vi "Auto 9.vi"(8 "Error In":errorcluster) -> (0 "Error Out":errorcluster)   [LabVIEW 2014]
uses:
  <vilib>/Rock Robotics/Network Tables/SD Read Boolean.vi
  Global Variables/Refnum Names.vi
  <vilib>/Rock Robotics/Network Tables/SD Read Number.vi
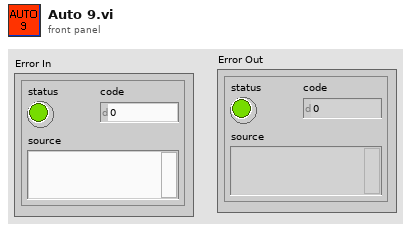
[diagram p1: front panel]
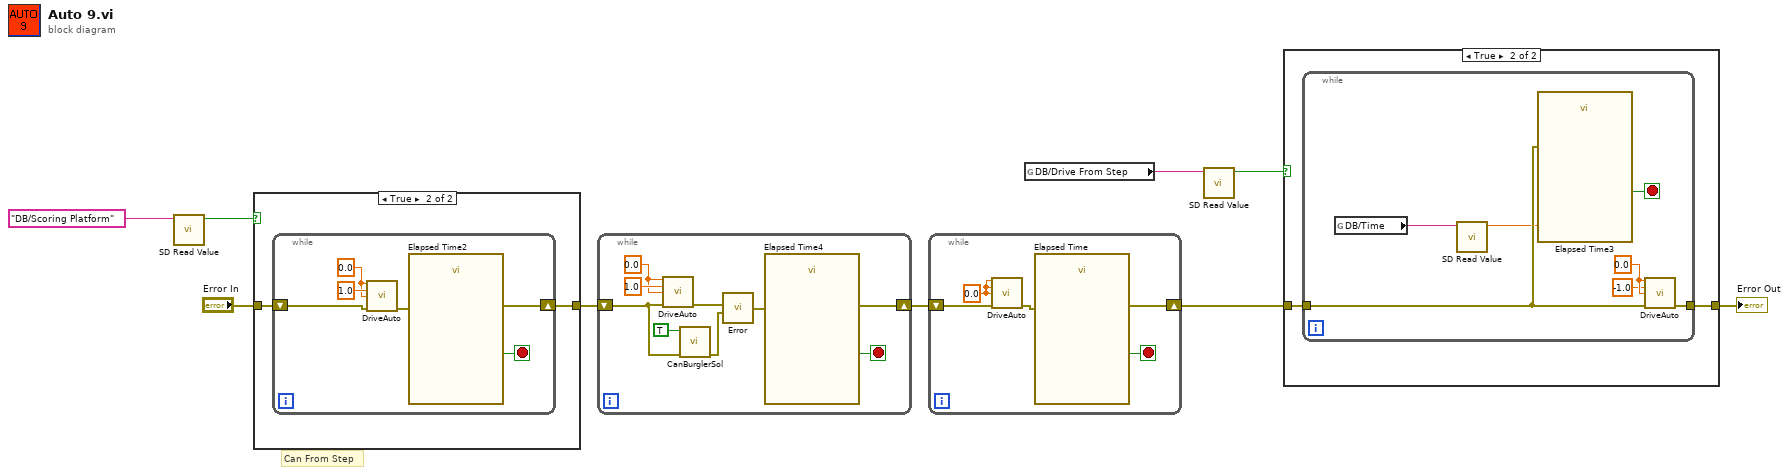
[diagram p0: block diagram]
diagram:
  # "Can From Step"
  n1 = call-poly <vilib>:"SD Read Value.vi"("Name"="DB/Scoring Platform") -> ("Boolean"=w4:bool)  [unwired: 8 in, 2 out]
  n2 = case shown="True" w4 {
    tunnel: "Error In" -> [w10 w11]
    tunnel: [w10 w12] -> w2
    frame False {
    }
    frame True {
      n3 = while {
        shift-right: [w14] -> w12
        shift-left: w11 -> [w15]
        stop <- w18 stop-if-true
        w16 = 0.0 ("Arm Value")
        n4 = call "DriveAuto.vi"("X In"=w16, "Y In"=1.0 ("X In"), "R In"=w16, "Error In"=w15) -> ("Error Out"=w13:errorcluster)  [unwired: 11 in]
        n5 = call "Elapsed Time2"("error in (no error)"=w13) -> ("Time has Elapsed"=w18:bool, "error out"=w14:errorcluster)  [unwired: 11 in, 6 out]
      }
    }
  }
  n6 = while {
    shift-right: [w23] -> w3
    shift-left: w2 -> [w24]
    stop <- w27 stop-if-true
    w25 = 0.0 ("Arm Value")
    n7 = call "DriveAuto.vi"("X In"=w25, "Y In"=1.0 ("X In"), "R In"=w25, "Error In"=w24) -> ("Error Out"=w22:errorcluster)  [unwired: 11 in]
    n8 = call "CanBurglerSol.vi"("Error In"=w24, "Grabber Open/Close"=TRUE) -> ("Error Out"=w21:errorcluster)  [unwired: 9 in]
    n9 = call "Error.vi"("error in (no error)"=w21, "error in (no error) 2"=w22) -> ("error out"=w20:errorcluster)  [unwired: 2 in]
    n10 = call "Elapsed Time4"("error in (no error)"=w20) -> ("Time has Elapsed"=w27:bool, "error out"=w23:errorcluster)  [unwired: 11 in, 6 out]
  }
  n11 = while {
    shift-right: [w30] -> w7
    shift-left: w3 -> [w31]
    stop <- w32 stop-if-true
    w28 = 0.0 ("Arm Value")
    n12 = call "DriveAuto.vi"("X In"=w28, "Y In"=w28, "R In"=w28, "Error In"=w31) -> ("Error Out"=w29:errorcluster)  [unwired: 11 in]
    n13 = call "Elapsed Time"("error in (no error)"=w29) -> ("Time has Elapsed"=w32:bool, "error out"=w30:errorcluster)  [unwired: 11 in, 6 out]
  }
  n14 = global read "Refnum Names.vi" "DB/Drive From Step"() -> (w1:string)
  n15 = call-poly <vilib>:"SD Read Value.vi"("Name"=w1) -> ("Boolean"=w6:bool)  [unwired: 8 in, 2 out]
  n16 = case shown="True" w6 {
    tunnel: w7 -> [w33 w35]
    tunnel: [w33 w34] -> w9
    frame False {
    }
    frame True {
      n17 = while {
        tunnel: [w42] -> w34
        tunnel: w35 -> [w39]
        stop <- w40 stop-if-true
        w41 = 0.0 ("Arm Value")
        n18 = global read "Refnum Names.vi" "DB/Time"() -> (w36:string)
        n19 = call-poly <vilib>:"SD Read Value.vi"("Name"=w36) -> ("Numeric"=w38:dbl)  [unwired: 8 in, 2 out]
        n20 = call "Elapsed Time3"("Time Target (s)"=w38, "error in (no error)"=w39) -> ("Time has Elapsed"=w40:bool)  [unwired: 10 in, 7 out]
        n21 = call "DriveAuto.vi"("X In"=w41, "Y In"=-1.0 ("X In"), "R In"=w41, "Error In"=w39) -> ("Error Out"=w42:errorcluster)  [unwired: 11 in]
      }
    }
  }
  "Error Out" <- w9
